vi "filtr_b.vi"(8 "threshold":i32=1, 11 "input array":dbl[][](array[numeric])) -> (3 "output array":dbl[][](array[numeric]))   [LabVIEW 2020]
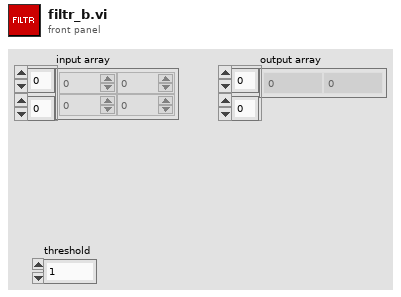
[diagram p1: front panel]
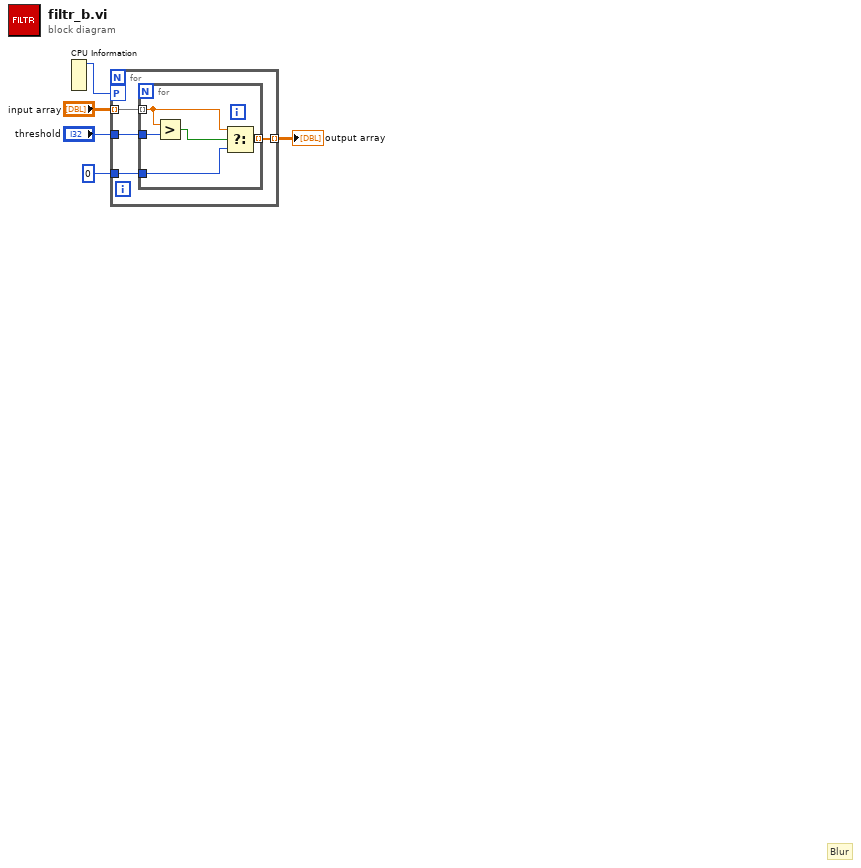
[diagram p0: block diagram]
diagram:
  # "Blur"
  n1 = CPU Information() -> (4:w1:i32)  [unwired: 3 out]
  n2 = for {
    tunnel: "input array" -> [w9] mode=indexing
    tunnel: "threshold" -> [w8]
    tunnel: [w7] -> w3 mode=indexing
    workers-P: w1 -> [_]
    tunnel: 0 -> [w6]
    n3 = for {
      tunnel: w9 -> [w12] mode=indexing
      tunnel: w8 -> [w11]
      tunnel: [w13] -> w7 mode=indexing
      tunnel: w6 -> [w14]
      n4 = Greater?(x=w12, y=w11) -> (0:w10:bool)
      n5 = Select(t=w12, s=w10, f=w14) -> (s? t:f=w13:dbl)
    }
  }
  "output array" <- w3
